vi "MGCC_StaEst_main_RTDS.vi"() -> ()   [LabVIEW 2016]
doc: "This VI is designed for the state estimation function block. The current version is designed for IEEE13node system. The advanced model will be available in the latest version. There is no input for this VI. Bascially, the input right now comes from the cvs in IEEE13 folder."
panel:
  in  "vbase":dbl=6928.4
  out "index":i32
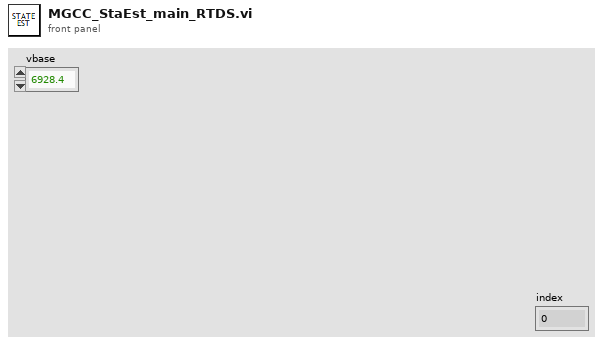
[diagram p1: front panel]
types:
  T1 = cluster{"V_node":cdb[][], "P_node":cdb[][], "I_node":cdb[][], "NumN":dbl, "NumL":dbl, "Ybus":cdb[][], "sspn":dbl[][], "ssqn":dbl[][], "ssvn":dbl[][], "SlackBus":dbl, "Topology":dbl[][]}
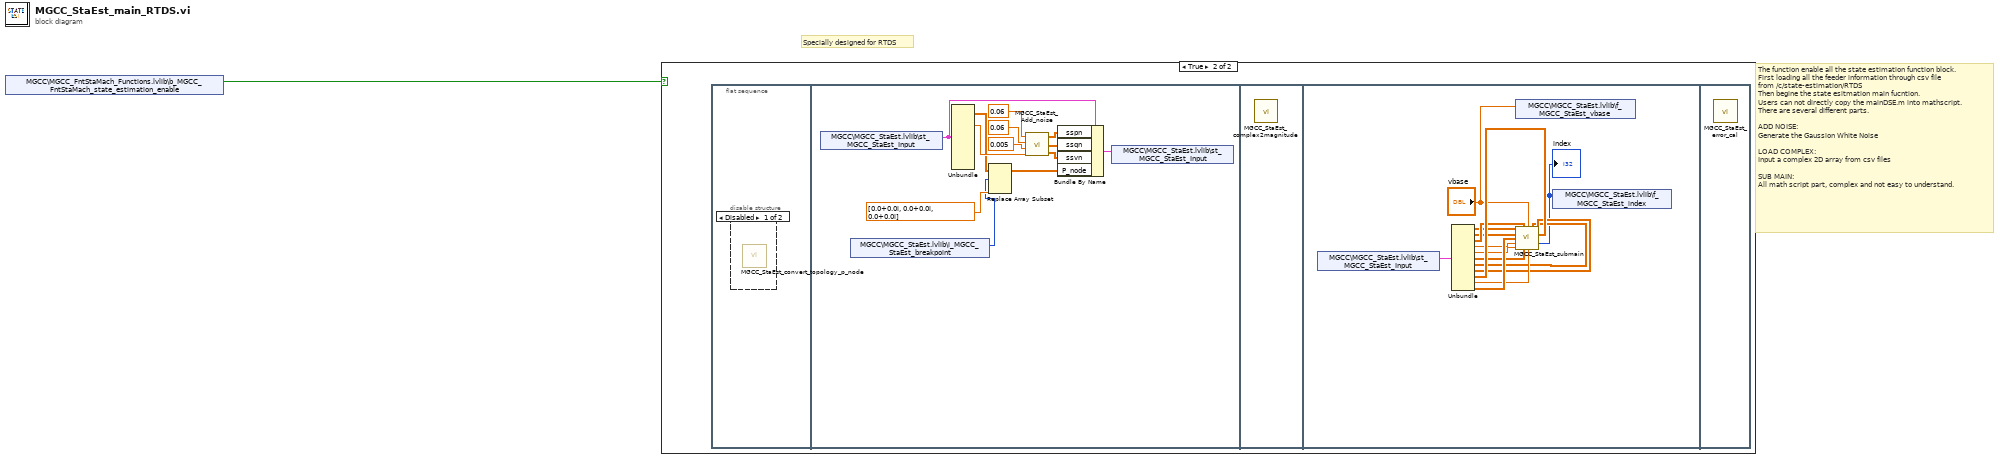
[diagram p0: block diagram]
diagram:
  # "Specially designed for RTDS"
  # "The function enable all the state estimation function block.\nFirst loading all the feeder information through csv file\nfrom /c/state-estimation/RTDS\nThen begine the state esitmation main fucntion.\nUsers can not directly copy the mainDSE.m into mathscript.\nThere are several different parts.\n\nADD NOISE:\nGenerate the Gaussion White Noise\n\nLOAD COMPLEX:\nInput a complex 2D array from csv files\n\nSUB MAIN:\nAll math script part, complex and not easy to understand."
  n1 = shared-variable "MGCC\\MGCC_FntStaMach_Functions.lvlib\\b_MGCC_FntStaMach_state_estimation_enable"() -> (w1:bool)  [unwired: 1 in, 1 out]
  n2 = case shown="True" w1 {
    frame False {
    }
    frame True {
      n3 = flat-sequence {
        frame #0 {
          n4 = disable-structure shown="Disabled" {
            frame Disabled {
              n5 = call "MGCC_StaEst_convert_topology_p_node.vi"() -> ()  [unwired: 12 in]
            }
            frame Enabled {
            }
          }
        }
        frame #1 {
          n6 = shared-variable "MGCC\\MGCC_StaEst.lvlib\\st_MGCC_StaEst_Input"() -> (w7:T1)  [unwired: 1 in, 1 out]
          n7 = shared-variable "MGCC\\MGCC_StaEst.lvlib\\i_MGCC_StaEst_breakpoint"() -> (w2:i32)  [unwired: 1 in, 1 out]
          n8 = Unbundle(w7) -> ("P_node"=w5:cdb[][], "NumN"=w6:dbl)  [unwired: 9 out]
          n9 = Replace Array Subset(array=w5, new element=cdb[] [0.0+0.0i, 0.0+0.0i, 0.0+0.0i] ("new element/subarray"), index (row)=w2) -> (w4:cdb[][])  [unwired: 1 in]
          n10 = call "MGCC_StaEst_Add_noise.vi"("Node"=w6, "svn"=0.005, "sqn"=0.06, "spn"=0.06) -> ("ssvn"=w8:dbl[][], "ssqn"=w9:dbl[][], "sspn"=w10:dbl[][])
          n11 = Bundle By Name(cluster=w7, "sspn"=w10, "ssqn"=w9, "ssvn"=w8, "P_node"=w4) -> (w14:T1)
          n12 = shared-variable "MGCC\\MGCC_StaEst.lvlib\\st_MGCC_StaEst_Input"(w14) -> ()  [unwired: 1 in, 1 out]
        }
        frame #2 {
          n13 = call "MGCC_StaEst_complex2magnitude.vi"() -> ()  [unwired: 12 in]
        }
        frame #3 {
          n14 = shared-variable "MGCC\\MGCC_StaEst.lvlib\\st_MGCC_StaEst_Input"() -> (w28:T1)  [unwired: 1 in, 1 out]
          n15 = Unbundle(w28) -> ("V_node"=w17:cdb[][], "P_node"=w18:cdb[][], "I_node"=w19:cdb[][], "NumN"=w20:dbl, "NumL"=w21:dbl, "Ybus"=w22:cdb[][], "sspn"=w23:dbl[][], "ssqn"=w24:dbl[][], "ssvn"=w25:dbl[][], "SlackBus"=w26:dbl, "Topology"=w27:dbl[][])
          n16 = shared-variable "MGCC\\MGCC_StaEst.lvlib\\f_MGCC_StaEst_vbase"("vbase") -> ()  [unwired: 1 in, 1 out]
          n17 = call "MGCC_StaEst_submain.vi"("V_node"=w17, "I_node"=w19, "vbase"="vbase", "sspn"=w23, "ssqn"=w24, "P_node"=w18, "ssvn"=w25, "Topology"=w27, "NumN"=w20, "NumL"=w21, "Ybus"=w22, "SlackBus"=w26) -> ("index"=w16:i32)  [unwired: 1 in, 2 out]
          "index" <- w16
          n18 = shared-variable "MGCC\\MGCC_StaEst.lvlib\\f_MGCC_StaEst_index"(w16) -> ()  [unwired: 1 in, 1 out]
        }
        frame #4 {
          n19 = call "MGCC_StaEst_error_cal.vi"() -> ()  [unwired: 12 in]
        }
      }
    }
  }
